vi "Nikhil_cmb1.vi"() -> ()   [LabVIEW 2014]
uses:
  <vilib>/addons/Digital Filter Design/Design.llb/DFD IIR Notch Peak Design by BW.vi
  <vilib>/addons/Digital Filter Design/Process.llb/DFD Filtering (Wfm NChan).vi
  <vilib>/addons/Digital Filter Design/NI_DigFilterLicensed.lvlib
panel:
  in  "stop (F)":bool
  out "Filtered Signal":dynamicdata(graph)
  out "Filtered Signal 2":dynamicdata(graph) caption="Filtered Signal"
  out "Filtered Signal 3":dynamicdata(graph) caption="Filtered Signal"
  out "Result":dynamicdata(graph)
  out "Result 3":dbl
  out "Amplitude":dbl
  out "Filtered Signal 4":dynamicdata(graph) caption="Filtered Signal"
  out "Boolean 2":bool
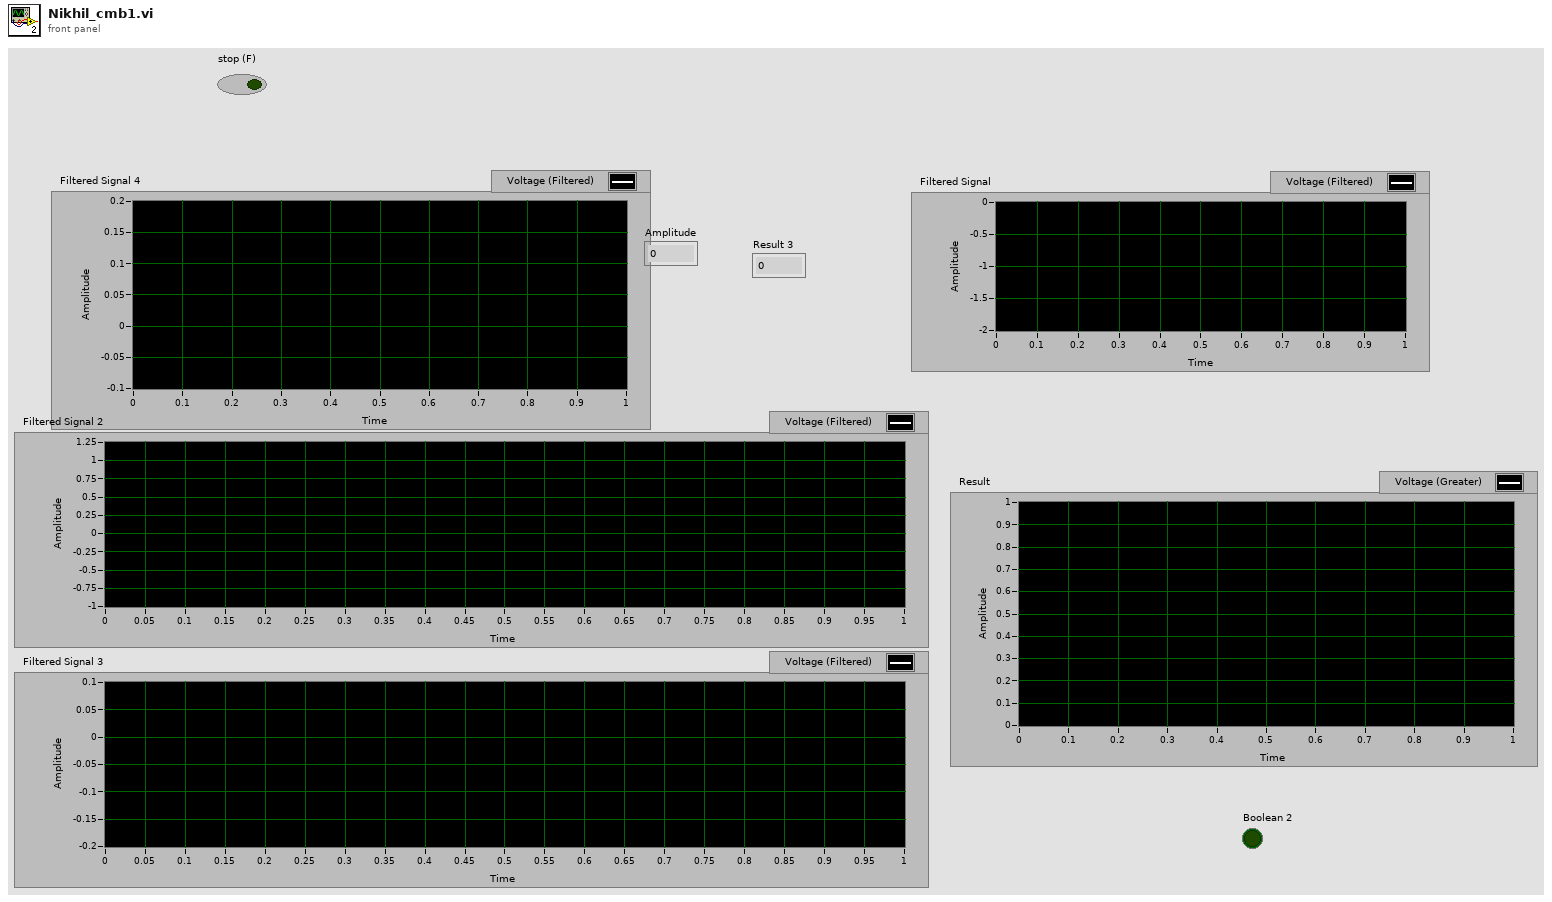
[diagram p1: front panel]
types:
  T1 = typedef "NI_DigFilterLicensed.lvlib/DFD Filter Obj.ctl" = cluster{"mSRate_Fs":dbl, "mSRate_Version":string, "mSRate_Comments":string, "mSRate_OrgCoef":T2, "mSRate_CurCoef":T2, "mSRate_Quantized?":bool, "mSRate_QCoef":T2, "mSRate_QSettings":T4[], "mSRate_Order":i32, "mSRate_Scaling":cluster{"mSRate_ScaleByPowerOf2?":bool, "mSRate_ScaleType":T6}}
  T2 = typedef "NI_DigFilterLicensed.lvlib/DFD Filter Coef.ctl" = cluster{"type":T3, "gain":dbl, "coef a (k)":dbl[], "coef b (v)":dbl[]}
  T3 = typedef "NI_DigFilterLicensed.lvlib/DFD Filter Structure Type Selector.ctl" = enum16{"Undefined", "FIR Direct Form", "FIR Direct Form Transposed", "FIR Symmetric", "FIR Antisymmetric", "IIR Direct Form I", "IIR Direct Form I Transposed", "IIR Direct Form II", "IIR Direct Form II Transposed", "IIR Cascaded Second Order Sections Form I", "IIR Cascaded Second Order Sections Form I Transposed", "IIR Cascaded Second Order Sections Form II", "IIR Cascaded Second Order Sections Form II Transposed", "Lattice Allpass (basic sections)", "Lattice Allpass (one multiplier sections)", "Lattice Allpass (normalized sections)", "Lattice AR (basic sections)", "Lattice AR (one multiplier sections)", "Lattice AR (normalized sections)", "Lattice MA (minimum phase)", "Lattice MA (maximum phase)", "Lattice ARMA (basic sections)", "Lattice ARMA (one multiplier sections)", "Lattice ARMA (normalized sections)"}
  T4 = typedef "NI_DigFilterLicensed.lvlib/dfd_Internal Quantization Settings.ctl" = cluster{"source":T5, "wl":i16, "iwl":i16, "overflow mode":enum16{"Saturation", "Wrap"}, "rounding mode":enum16{"Nearest", "Truncation"}, "signed?":bool}
  T5 = typedef "NI_DigFilterLicensed.lvlib/dfd_Internal Quantization Srcs.ctl" = u16
  T6 = typedef "NI_DigFilterLicensed.lvlib/DFD Coef Norm Type.ctl" = enum16{"No Norm", "Time Domain 1-Norm", "Time Domain 2-Norm", "Time Domain Inf-Norm"}
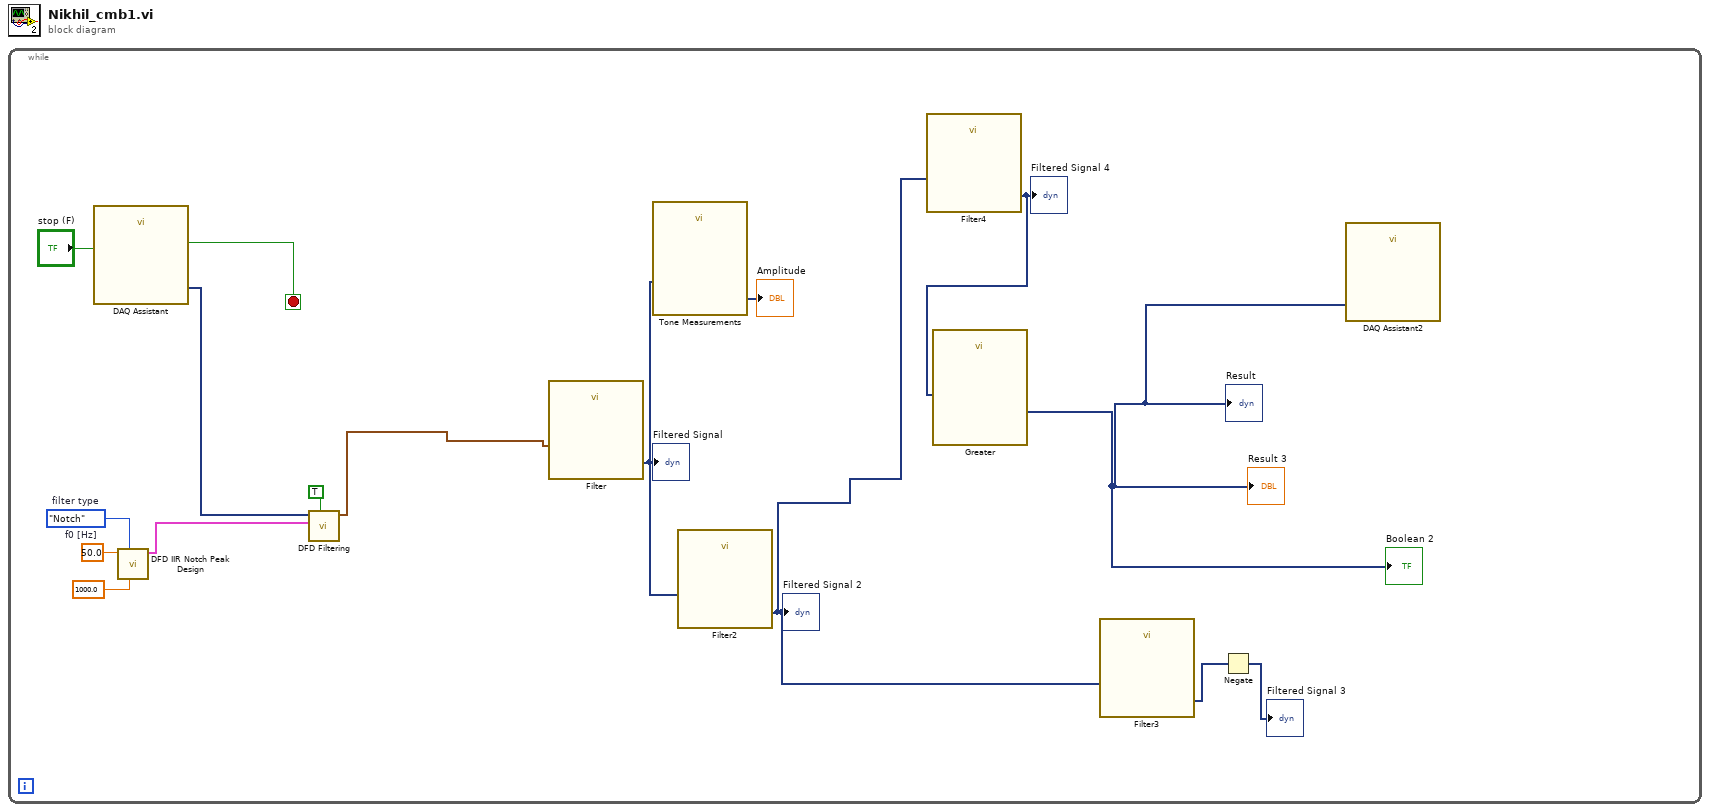
[diagram p0: block diagram]
diagram:
  n1 = while {
    stop <- w15 stop-if-true
    w7 = enum16{"Notch", "Peak"}."Notch"  # filter type
    w9 = 50.0  # f0 [Hz]
    n2 = call "DAQ Assistant"("stop (F)"="stop (F)") -> ("data"=w5:dynamicdata, "stopped"=w15:bool)  [unwired: 15 in, 2 out]
    n3 = call-poly <vilib>:"DFD IIR Notch Peak Design.vi"("fs [Hz]"=1000.0, "filter type"=w7, "f0 [Hz]"=w9) -> ("filter out"=w6:T1)  [unwired: 3 in, 5 out]
    n4 = call-poly <vilib>:"DFD Filtering.vi"("init? (F)"=TRUE, "filter"=w6, "signal in"=w5) -> ("signal out"=w4:waveform(dbl)[])  [unwired: 1 in, 7 out]
    n5 = call "Filter"("Signal"=w4) -> ("Filtered Signal"=w3:dynamicdata)  [unwired: 9 in, 1 out]
    "Filtered Signal" <- w3
    n6 = call "Tone Measurements"("Signals"=w3) -> ("Amplitude"=→"Amplitude":dynamicdata)  [unwired: 9 in, 1 out]
    n7 = call "Filter2"("Signal"=w3) -> ("Filtered Signal"=w10:dynamicdata)  [unwired: 9 in, 1 out]
    "Filtered Signal 2" <- w10
    n8 = call "Filter4"("Signal"=w10) -> ("Filtered Signal"=w1:dynamicdata)  [unwired: 9 in, 1 out]
    "Filtered Signal 4" <- w1
    n9 = call "Greater"("Operand 1"=w1) -> ("Result"=w11:dynamicdata)  [unwired: 9 in, 1 out]
    "Result" <- w11
    "Result 3" <- w11
    "Boolean 2" <- w11
    n10 = call "Filter3"("Signal"=w10) -> ("Filtered Signal"=w14:dynamicdata)  [unwired: 9 in, 1 out]
    n11 = Negate(x=w14) -> (-x=→"Filtered Signal 3":dynamicdata)
    n12 = call "DAQ Assistant2"("data"=w11) -> ()  [unwired: 16 in, 3 out]
  }
